vi "Untitled 5.vi"() -> ()   [LabVIEW 2015]
panel:
  out "All Tags":string[](array[string])
  in  "Tree":string(tree)
  out "Number of Rows":u32
  out "Value":i32
  in  "Used Channels":i32(listbox)
  in  "Ring":u16(ring)
  in  "DevNames":tag[](array[tag])
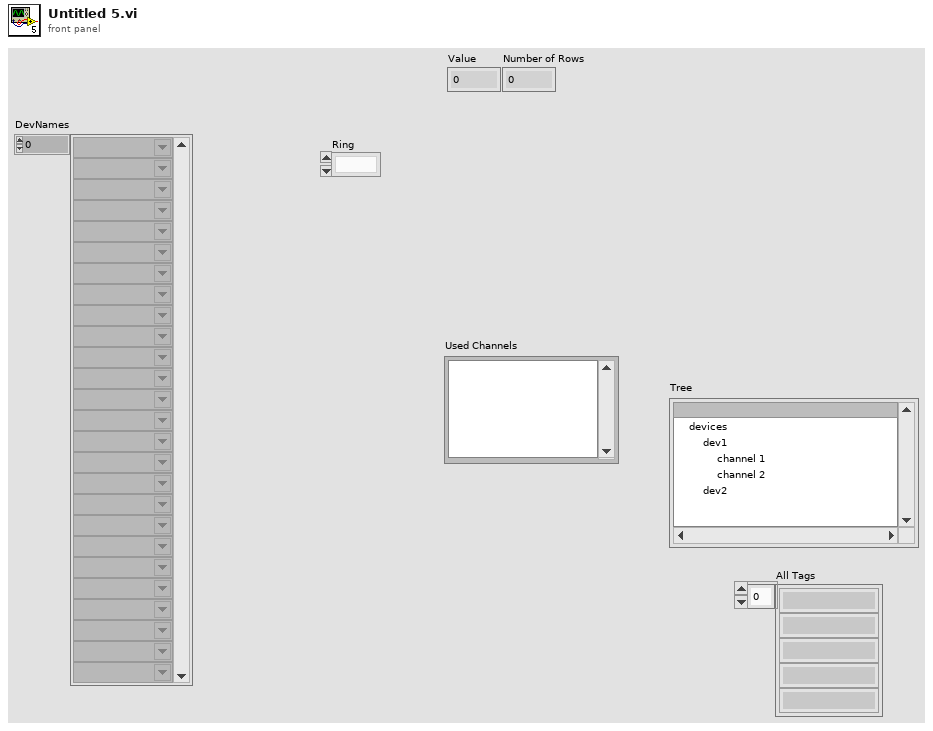
[diagram p1: front panel]
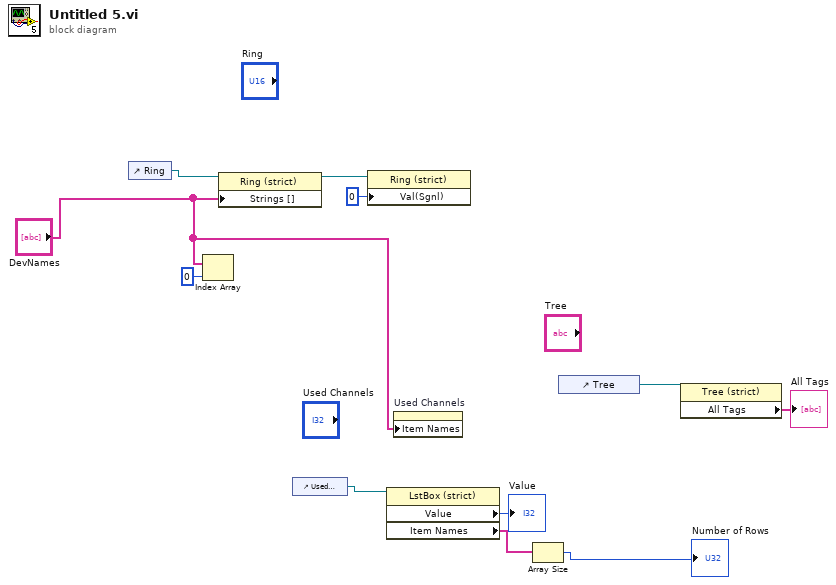
[diagram p0: block diagram]
diagram:
  n1 = control-ref of="Ring"() -> (w11:refnum<vi>)
  n2 = Index Array(array="DevNames", index=0) -> ()  [unwired: 1 out]
  n3 = property class="Ring (strict)"(reference=w11, "Strings []"="DevNames") -> (reference out=w10:refnum<vi>)  [unwired: 1 in, 1 out]
  n4 = control-ref of="Used Channels"() -> (w6:refnum<vi>)
  n5 = property class="Ring (strict)"(reference=w10, "Val(Sgnl)"=u16 0 ("Value")) -> ()  [unwired: 1 in, 2 out]
  n6 = property on="Property Node" class="LstBox (strict)"(reference=w6) -> ("Value"=→"Value":i32, "Item Names"=w4:string[])  [unwired: 1 in, 2 out]
  n7 = property on="Used Channels" class="LstBox (strict)"("Item Names"="DevNames") -> ()  [unwired: 2 in, 2 out]
  n8 = Array Size(array=w4) -> (size(s)=→"Number of Rows":i32)
  n9 = control-ref of="Tree"() -> (w2:refnum<vi>)
  n10 = property on="Property Node" class="Tree (strict)"(reference=w2) -> ("All Tags"=→"All Tags":string[])  [unwired: 1 in, 2 out]
